vi "Read Rule list.vi"(11 "CRuleList in":refnum<class "CRuleList.lvclass">) -> (2 "Rule List":T1, 3 "CRuleList out":refnum<class "CRuleList.lvclass">)   [LabVIEW 2020, in "DependencyInspection.lvlib" / "CRuleList.lvclass"]
uses:
  CRuleList.lvclass
  RuleList.ctl
  obj/Addons/LabVIEWObjectInterfaces.lvlibp/LabVIEWObjectInterfaces/IDependencyItemRule/IDependencyItemRule.lvclass
  CRuleList.lvclass/CRuleList.ctl
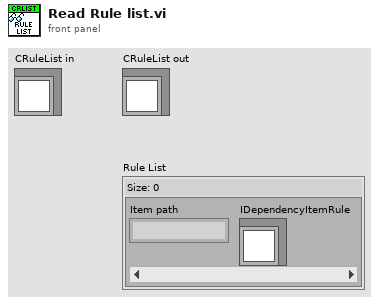
[diagram p1: front panel]
types:
  T1 = typedef "DependencyInspection.lvlib/CRuleList.lvclass/RuleList.ctl" = map{string, refnum<class "IDependencyItemRule.lvclass">}
  T2 = typedef "DependencyInspection.lvlib/CRuleList.lvclass/RuleListRef.ctl" = refnum<data-value>
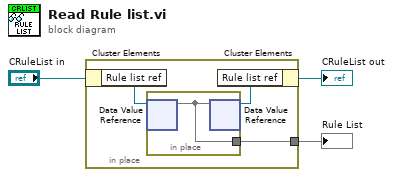
[diagram p0: block diagram]
diagram:
  n1 = in-place {
    in-place-border: [w6] -> w1
    n2 = in-place-cluster #1("CRuleList in") -> ("Rule list ref"=w5:T2)
    n3 = in-place {
      in-place-border: [w7] -> w6
      n4 = in-place-dvr #2(w5) -> (w7:T1)  [unwired: 1 out]
      n5 = in-place-dvr #2(w7) -> (w4:T2)  [unwired: 1 out]
    }
    n6 = in-place-cluster #1("Rule list ref"=w4) -> (→"CRuleList out":refnum<class "CRuleList.lvclass">)
  }
  "Rule List" <- w1
